vi "OLA.vi"() -> ()   [LabVIEW 2019]
doc: "This is the On-Line Analysis module (OLA).\nThis module receives events from the Target Event Builder (TEB) and processes them. The Q Curve is massaged, gains are divided out, the subtracted and poly subtracted signals are calculated, and an area measurement is made. These results are then sent to the Polarization Display Panel (PDP)."
panel:
  out "data_ready":bool
  out "status":string
  in  "port":u16=10000
  out "Bottom Charge":dbl format="%.6e"
  out "Top Charge":dbl format="%.6e"
  in  "Previous Event":i32
  in  "stop":bool
  out "RF Mod":i32
  out "RF Freq":dbl format="%.3f"
  out "Cal Const":dbl format="%.6f"
  out "Baseline":i32
  out "Raw Signal":dbl[](array[numeric]) format="%.4f"
  out "Event Number":i32
  out "Area":dbl format="%.6f"
  out "Polarization":dbl format="%.2f"
  out "PolySubtracted Signal":dbl[](array[numeric]) format="%.4f"
  out "Polyfit Curve":dbl[](array[numeric]) format="%.4f"
  out "Subtracted Signal":dbl[](array[numeric]) format="%.4f"
  out "Baseline Signal":dbl[](array[numeric]) format="%.6f"
  # "Params over TCP/IP"
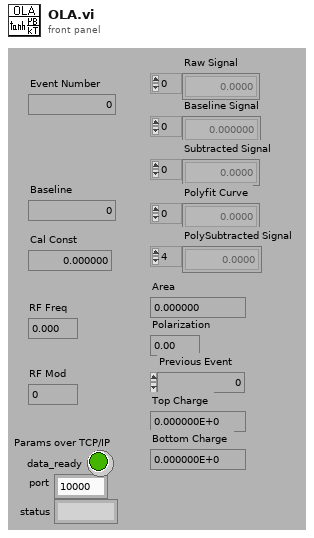
[diagram p1: front panel]
types:
  T1 = enum16{"No Message", "Bad Message", "ClearCharge", "Event=", "Address=", "Ping=", "Stop"}
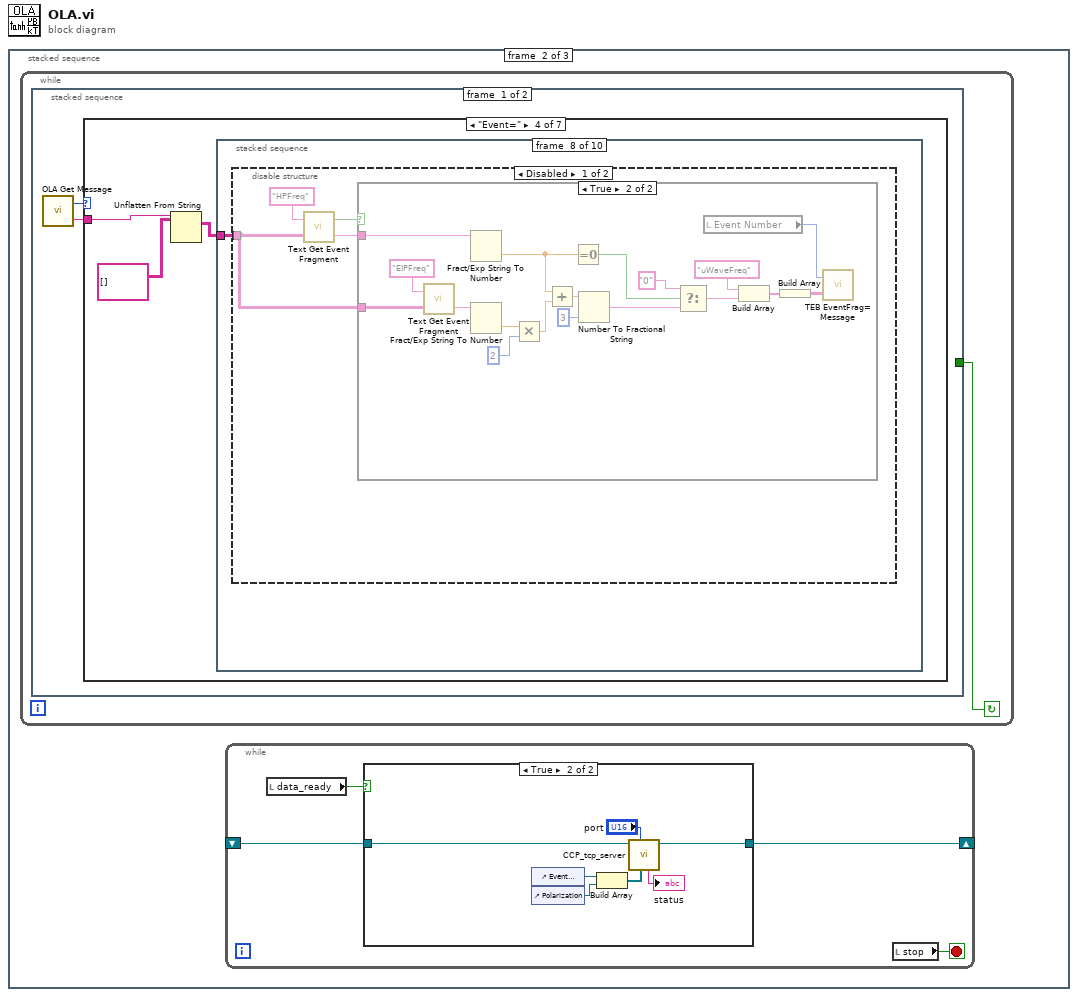
[diagram p0: block diagram]
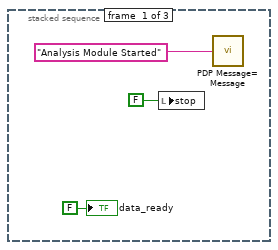
[diagram p2: hidden frame]
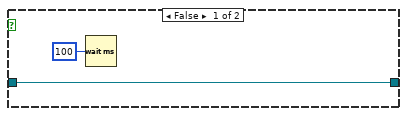
[diagram p3: hidden frame]
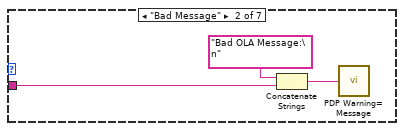
[diagram p5: hidden frame]
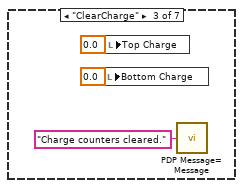
[diagram p6: hidden frame]
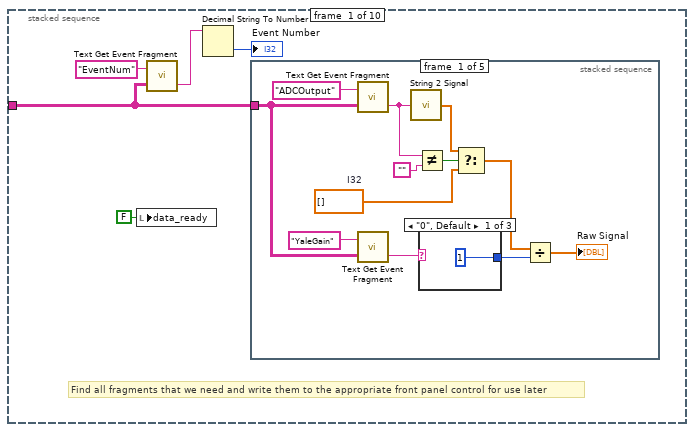
[diagram p7: hidden frame]
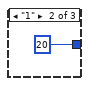
[diagram p8: hidden frame]
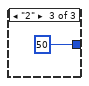
[diagram p9: hidden frame]
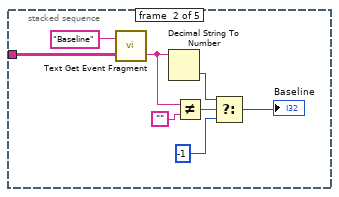
[diagram p10: hidden frame]
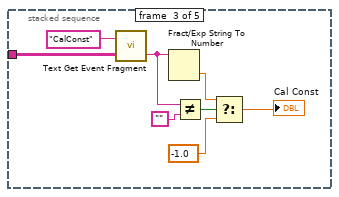
[diagram p11: hidden frame]
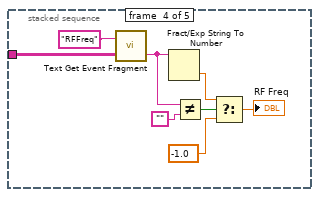
[diagram p12: hidden frame]
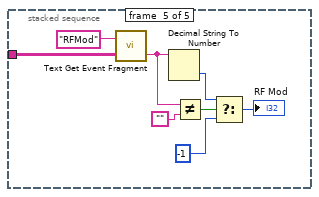
[diagram p13: hidden frame]
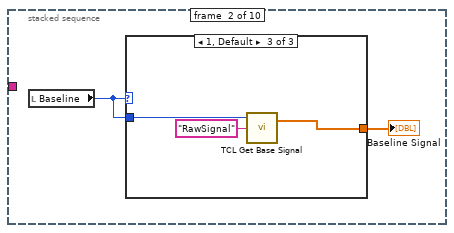
[diagram p14: hidden frame]
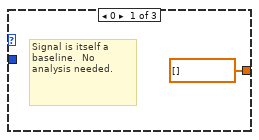
[diagram p15: hidden frame]
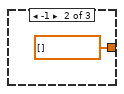
[diagram p16: hidden frame]
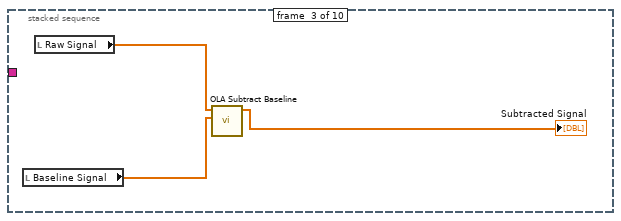
[diagram p17: hidden frame]
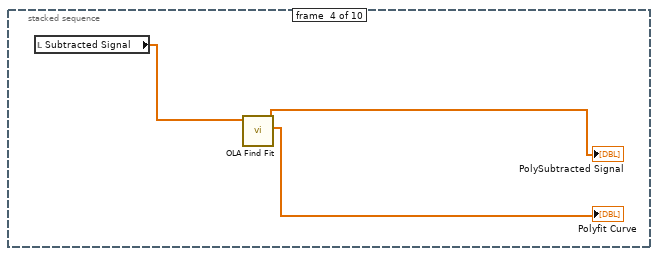
[diagram p18: hidden frame]
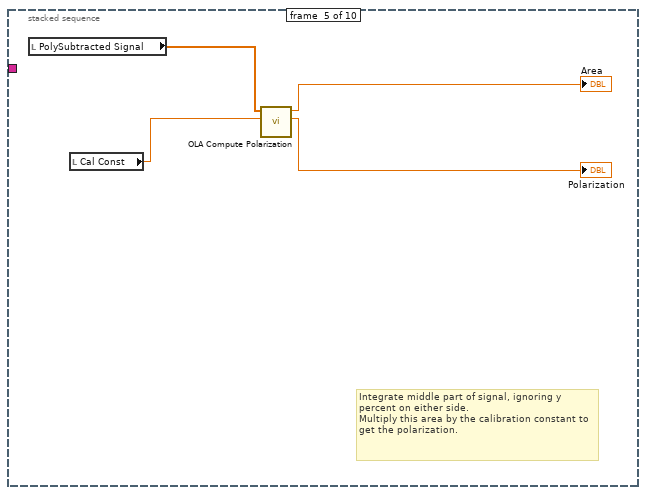
[diagram p19: hidden frame]
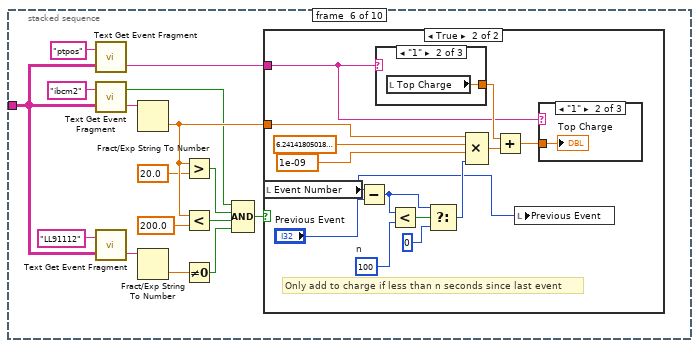
[diagram p20: hidden frame]
diagram:
  n1 = stacked-sequence {
    frame #0 {
      n2 = local write "stop"(FALSE ("stop")) -> ()
      n3 = call "PDP Message= Message.vi"("Message"="Analysis Module Started") -> ()
      "data_ready" <- FALSE ("data_ready")
    }
    frame #1 {
      n4 = while {
        stop <- w17 continue-if-true
        n5 = stacked-sequence {
          tunnel: [_ w238] -> w17
          frame #0 {
            n6 = call "OLA Get Message.vi"() -> ("Text"=w19:string, "OLA Message Type"=w18:T1)
            n7 = case shown="\"Event=\"" w18 {
              tunnel: w19 -> [_ w22 _ w27 w230 w233 _]
              frame "No Message" {
              }
              frame "Bad Message" {
                n8 = Concatenate Strings("Bad OLA Message:\n", w22) -> (w20:string)
                n9 = call "PDP Warning= Message.vi"("Message"=w20) -> ()
              }
              frame "ClearCharge" {
                n10 = local write "Bottom Charge"(0.0 ("Bottom Charge")) -> ()
                n11 = local write "Top Charge"(0.0 ("Top Charge")) -> ()
                n12 = call "PDP Message= Message.vi"("Message"="Charge counters cleared.") -> ()
              }
              frame "Event=" {
                (unwired) FALSE
                n13 = Unflatten From String(type=string[][] [], binary string=w27) -> (value=w26:string[][])  [unwired: 3 in, 2 out]
                n14 = stacked-sequence {
                  tunnel: w26 -> [w30 _ _ _ _ w101 w134 w151 _ _]
                  frame #0 {
                    # "Find all fragments that we need and write them to the appropriate front panel control for use later"
                    n15 = local write "data_ready"(FALSE ("data_ready")) -> ()
                    n16 = call "Text Get Event Fragment.vi"("Event"=w30, "Fragment Type"="EventNum") -> ("Fragment"=w32:string)  [unwired: 1 out]
                    n17 = Decimal String To Number(string=w32) -> (number=→"Event Number":i32)  [unwired: 2 in, 1 out]
                    n18 = stacked-sequence {
                      tunnel: w30 -> [w39 w55 w63 w71 w79]
                      frame #0 {
                        w34 = dbl[] []  # I32
                        n19 = call "Text Get Event Fragment.vi"("Event"=w39, "Fragment Type"="ADCOutput") -> ("Fragment"=w44:string)  [unwired: 1 out]
                        n20 = call "Text Get Event Fragment.vi"("Event"=w39, "Fragment Type"="YaleGain") -> ("Fragment"=w38:string)  [unwired: 1 out]
                        n21 = call "String 2 Signal.vi"("String"=w44) -> ("Signal"=w41:dbl[])
                        n22 = Not Equal?(x=w44, y="") -> (x != y?=w43:bool)
                        n23 = case shown="\"0\", Default" w38 {
                          tunnel: [1 20 50] -> w37
                          frame "0", Default {
                          }
                          frame "1" {
                          }
                          frame "2" {
                          }
                        }
                        n24 = Select(t=w41, s=w43, f=w34) -> (s? t:f=w36:dbl[])
                        n25 = Divide(x=w36, y=w37) -> (x/y=→"Raw Signal":dbl[])
                      }
                      frame #1 {
                        n26 = call "Text Get Event Fragment.vi"("Event"=w55, "Fragment Type"="Baseline") -> ("Fragment"=w50:string)  [unwired: 1 out]
                        n27 = Decimal String To Number(string=w50) -> (number=w53:i32)  [unwired: 2 in, 1 out]
                        n28 = Not Equal?(x=w50, y="") -> (x != y?=w52:bool)
                        n29 = Select(t=w53, s=w52, f=-1) -> (s? t:f=→"Baseline":i32)
                      }
                      frame #2 {
                        n30 = call "Text Get Event Fragment.vi"("Event"=w63, "Fragment Type"="CalConst") -> ("Fragment"=w58:string)  [unwired: 1 out]
                        n31 = Fract/Exp String To Number(string=w58) -> (number=w61:dbl)  [unwired: 3 in, 1 out]
                        n32 = Not Equal?(x=w58, y="") -> (x != y?=w60:bool)
                        n33 = Select(t=w61, s=w60, f=-1.0) -> (s? t:f=→"Cal Const":dbl)
                      }
                      frame #3 {
                        n34 = call "Text Get Event Fragment.vi"("Event"=w71, "Fragment Type"="RFFreq") -> ("Fragment"=w66:string)  [unwired: 1 out]
                        n35 = Fract/Exp String To Number(string=w66) -> (number=w69:dbl)  [unwired: 3 in, 1 out]
                        n36 = Not Equal?(x=w66, y="") -> (x != y?=w68:bool)
                        n37 = Select(t=w69, s=w68, f=-1.0) -> (s? t:f=→"RF Freq":dbl)
                      }
                      frame #4 {
                        n38 = call "Text Get Event Fragment.vi"("Event"=w79, "Fragment Type"="RFMod") -> ("Fragment"=w74:string)  [unwired: 1 out]
                        n39 = Decimal String To Number(string=w74) -> (number=w77:i32)  [unwired: 2 in, 1 out]
                        n40 = Not Equal?(x=w74, y="") -> (x != y?=w76:bool)
                        n41 = Select(t=w77, s=w76, f=-1) -> (s? t:f=→"RF Mod":i32)
                      }
                    }
                  }
                  frame #1 {
                    n42 = local read "Baseline"() -> (w82:i32)
                    n43 = case shown="1, Default" w82 {
                      tunnel: w82 -> [_ _ w87]
                      tunnel: [dbl[] [] ("Baseline") dbl[] [] ("Baseline") w86] -> w81
                      frame 0 {
                        # "Signal is itself a baseline.  No analysis needed."
                      }
                      frame -1 {
                      }
                      frame 1, Default {
                        n44 = call "TCL Get Base Signal.vi"("signal name"="RawSignal", "event number"=w87) -> ("signal"=w86:dbl[])  [unwired: 1 in, 1 out]
                      }
                    }
                    "Baseline Signal" <- w81
                  }
                  frame #2 {
                    n45 = local read "Baseline Signal"() -> (w89:dbl[])
                    n46 = local read "Raw Signal"() -> (w90:dbl[])
                    n47 = call "OLA Subtract Baseline.vi"("baseline"=w89, "raw"=w90) -> ("subtracted"=→"Subtracted Signal":dbl[])  [unwired: 9 in]
                  }
                  frame #3 {
                    n48 = local read "Subtracted Signal"() -> (w93:dbl[])
                    n49 = call "OLA Find Fit.vi"("signal"=w93) -> ("fit"=→"Polyfit Curve":dbl[], "subtracted"=→"PolySubtracted Signal":dbl[])  [unwired: 8 in, 1 out]
                  }
                  frame #4 {
                    # "Integrate middle part of signal, ignoring y percent on either side.\nMultiply this area by the calibration constant to get the polarization."
                    n50 = local read "PolySubtracted Signal"() -> (w97:dbl[])
                    n51 = local read "Cal Const"() -> (w96:dbl)
                    n52 = call "OLA Compute Polarization.vi"("cal"=w96, "signal"=w97) -> ("polarization"=→"Polarization":dbl, "area"=→"Area":dbl)  [unwired: 8 in]
                  }
                  frame #5 {
                    n53 = call "Text Get Event Fragment.vi"("Event"=w101, "Fragment Type"="ptpos") -> ("Fragment"=w99:string)  [unwired: 1 out]
                    n54 = call "Text Get Event Fragment.vi"("Event"=w101, "Fragment Type"="ibcm2") -> ("Fragment"=w110:string, "Found"=w98:bool)
                    n55 = call "Text Get Event Fragment.vi"("Event"=w101, "Fragment Type"="LL91112") -> ("Fragment"=w112:string)  [unwired: 1 out]
                    n56 = Fract/Exp String To Number(string=w110) -> (number=w109:dbl)  [unwired: 3 in, 1 out]
                    n57 = Fract/Exp String To Number(string=w112) -> (number=w111:dbl)  [unwired: 3 in, 1 out]
                    n58 = Greater?(x=w109, y=20.0) -> (0:w104:bool)
                    n59 = Less?(x=w109, y=200.0) -> (x < y?=w106:bool)
                    n60 = Not Equal To 0?(x=w111) -> (x != 0?=w105:bool)
                    n61 = Compound Arithmetic op=AND(w98, w104, w106, w105) -> (w103:bool)
                    n62 = case shown="True" w103 {
                      tunnel: w109 -> [_ w124]
                      tunnel: w99 -> [_ w115]
                      frame False {
                      }
                      frame True {
                        w123 = 100  # n
                        # "Only add to charge if less than n seconds since last event"
                        n63 = local read "Event Number"() -> (w114:i32)
                        n64 = Subtract(x=w114, y="Previous Event") -> (x-y=w120:i32)
                        n65 = case shown="\"1\"" w115 {
                          tunnel: [0.0 w131 w132] -> w117
                          frame "0", Default {
                          }
                          frame "1" {
                            n66 = local read "Top Charge"() -> (w131:dbl)
                          }
                          frame "2" {
                            n67 = local read "Bottom Charge"() -> (w132:dbl)
                          }
                        }
                        n68 = Less?(x=w120, y=w123) -> (x < y?=w121:bool)
                        n69 = Select(t=w120, s=w121, f=0) -> (s? t:f=w118:i32)
                        n70 = Compound Arithmetic op=MULTIPLY(w124, 6.241418050181001e+18, 1e-09 ("Input"), w118) -> (w122:dbl)
                        n71 = Add(x=w117, y=w122) -> (x+y=w116:dbl)
                        n72 = local write "Previous Event"(w114) -> ()
                        n73 = case shown="\"1\"" w115 {
                          tunnel: w116 -> [_ w128 w129]
                          frame "0", Default {
                          }
                          frame "1" {
                            "Top Charge" <- w128
                          }
                          frame "2" {
                            "Bottom Charge" <- w129
                          }
                        }
                      }
                    }
                  }
                  frame #6 {
                    n74 = call "Text Get Event Fragment.vi"("Event"=w134, "Fragment Type"="He4Temp") -> ("Found"=w133:bool)  [unwired: 1 out]
                    n75 = case shown="False" w133 {
                      tunnel: w134 -> [w142 _]
                      frame False {
                        n76 = call "Text Get Event Fragment.vi"("Event"=w142, "Fragment Type"="He4Press") -> ("Fragment"=w150:string)  [unwired: 1 out]
                        n77 = call "Text Get Event Fragment.vi"("Event"=w142, "Fragment Type"="He4Range") -> ("Fragment"=w141:string)  [unwired: 1 out]
                        n78 = Fract/Exp String To Number(string=w150) -> (number=w136:dbl)  [unwired: 3 in, 1 out]
                        n79 = Fract/Exp String To Number(string=w141) -> (number=w140:dbl)  [unwired: 3 in, 1 out]
                        n80 = expression code="10**(-x+2)"(w140) -> (w139:dbl)
                        n81 = Multiply(x=w136, y=w139) -> (x*y=w137:dbl)
                        n82 = call "TTM 4He Press to Temp.vi"("4He Vapor Pressure (torr)"=w137) -> ("4He Temp (K)"=w138:dbl)
                        n83 = Number To Exponential String(number=w138) -> (E-format string=w148:string)  [unwired: 3 in]
                        n84 = local read "Event Number"() -> (w145:i32)
                        n85 = Build Array("He4Temp", w148) -> (w144:string[])
                        n86 = Build Array(w144) -> (w146:string[][])
                        n87 = call "TEB EventFrag= Message.vi"("Event Fragment(s)"=w146, "Event Number"=w145) -> ()
                      }
                      frame True {
                      }
                    }
                  }
                  frame #7 {
                    n88 = disable-structure shown="Disabled" {
                      disable-tunnel: w151 -> [w154 _]
                      frame Disabled {
                        n89 = call "Text Get Event Fragment.vi"("Event"=w154, "Fragment Type"="HPFreq") -> ("Fragment"=w152:string, "Found"=w153:bool)
                        n90 = case shown="True" w153 {
                          tunnel: w154 -> [w157 w175]
                          tunnel: w152 -> [_ w172]
                          frame False {
                            n91 = call "Text Get Event Fragment.vi"("Event"=w157, "Fragment Type"="EIPFreq") -> ("Fragment"=w156:string)  [unwired: 1 out]
                            n92 = local read "Event Number"() -> (w159:i32)
                            n93 = Build Array("uWaveFreq", w156) -> (w158:string[])
                            n94 = Build Array(w158) -> (w160:string[][])
                            n95 = call "TEB EventFrag= Message.vi"("Event Fragment(s)"=w160, "Event Number"=w159) -> ()
                          }
                          frame True {
                            n96 = call "Text Get Event Fragment.vi"("Event"=w175, "Fragment Type"="EIPFreq") -> ("Fragment"=w174:string)  [unwired: 1 out]
                            n97 = Fract/Exp String To Number(string=w172) -> (number=w165:dbl)  [unwired: 3 in, 1 out]
                            n98 = Fract/Exp String To Number(string=w174) -> (number=w173:dbl)  [unwired: 3 in, 1 out]
                            n99 = Multiply(x=w173, y=2) -> (x*y=w171:dbl)
                            n100 = Add(x=w165, y=w171) -> (x+y=w170:dbl)
                            n101 = Equal To 0?(x=w165) -> (x = 0?=w164:bool)
                            n102 = Number To Fractional String(number=w170, precision (6)=i16 3) -> (F-format string=w166:string)  [unwired: 2 in]
                            n103 = Select(t="0", s=w164, f=w166) -> (s? t:f=w167:string)
                            n104 = local read "Event Number"() -> (w177:i32)
                            n105 = Build Array("uWaveFreq", w167) -> (w176:string[])
                            n106 = Build Array(w176) -> (w178:string[][])
                            n107 = call "TEB EventFrag= Message.vi"("Event Fragment(s)"=w178, "Event Number"=w177) -> ()
                          }
                        }
                      }
                      frame Enabled {
                      }
                    }
                  }
                  frame #8 {
                    w183 = string[] [] ("Array Constant")
                    # "Ship all results off to the event builder."
                    n108 = local read "PolySubtracted Signal"() -> (w181:dbl[])
                    n109 = local read "Bottom Charge"() -> (w193:dbl)
                    n110 = local read "Subtracted Signal"() -> (w218:dbl[])
                    n111 = local read "Polyfit Curve"() -> (w217:dbl[])
                    n112 = local read "Polarization"() -> (w204:dbl)
                    n113 = local read "Baseline Signal"() -> (w223:dbl[])
                    n114 = local read "Top Charge"() -> (w194:dbl)
                    n115 = local read "Raw Signal"() -> (w201:dbl[])
                    n116 = local read "Area"() -> (w212:dbl)
                    n117 = Array Size(array=w181) -> (size(s)=w182:i32)
                    n118 = Equal To 0?(x=w182) -> (x = 0?=w184:bool)
                    n119 = call "Signal 2 String.vi"("Signal"=w201) -> ("String"=w202:string)
                    n120 = call "Signal 2 String.vi"("Signal"=w223) -> ("String"=w222:string)
                    n121 = call "Signal 2 String.vi"("Signal"=w218) -> ("String"=w219:string)
                    n122 = call "Signal 2 String.vi"("Signal"=w217) -> ("String"=w216:string)
                    n123 = call "Signal 2 String.vi"("Signal"=w181) -> ("String"=w213:string)
                    n124 = Number To Exponential String(number=w194) -> (E-format string=w196:string)  [unwired: 3 in]
                    n125 = Number To Exponential String(number=w193) -> (E-format string=w191:string)  [unwired: 3 in]
                    n126 = Number To Exponential String(number=w204) -> (E-format string=w205:string)  [unwired: 3 in]
                    n127 = Number To Exponential String(number=w212) -> (E-format string=w211:string)  [unwired: 3 in]
                    n128 = Build Array("RawSignal", w202) -> (w200:string[])
                    n129 = Build Array("BaseSignal", w222) -> (w199:string[])
                    n130 = Build Array("SubSignal", w219) -> (w198:string[])
                    n131 = Build Array("PolyCurve", w216) -> (w197:string[])
                    n132 = Build Array("PolySignal", w213) -> (w209:string[])
                    n133 = Build Array("TopCharge", w196) -> (w190:string[])
                    n134 = Build Array("BottomCharge", w191) -> (w189:string[])
                    n135 = Build Array("Polarization", w205) -> (w188:string[])
                    n136 = Build Array("Area", w211) -> (w187:string[])
                    n137 = Select(t=w183, s=w184, f=w188) -> (s? t:f=w185:string[])
                    n138 = Select(t=w183, s=w184, f=w187) -> (s? t:f=w186:string[])
                    n139 = local read "Event Number"() -> (w207:i32)
                    n140 = Build Array(w200, w199, w198, w197, w209, w190, w189, w185, w186) -> (w208:string[][])
                    n141 = call "TEB EventFrag= Message.vi"("Event Fragment(s)"=w208, "Event Number"=w207) -> ()
                  }
                  frame #9 {
                    # "Tell event builder we're done processing this event."
                    n142 = local read "Event Number"() -> (w226:i32)
                    n143 = local write "data_ready"(TRUE ("data_ready")) -> ()
                    n144 = call "TEB Processed= Message.vi"("Module Name"="OLA", "Event Number"=w226) -> ()
                  }
                }
              }
              frame "Address=" {
                n145 = Scan From String(format string="%s,%[.0-9]:%d" ("Format String"), input string=w230) -> (output 1=w228:string, output 2=w229:string, output 3=w227:i32)  [unwired: 5 in, 3 out]
                n146 = call "Message Set Module Address.vi"("Port"=w227, "Address"=w229, "Module"=w228) -> ()
              }
              frame "Ping=" {
                n147 = Get Date/Time In Seconds() -> (seconds since 1Jan1904=w232:timestamp)
                n148 = To Double Precision Float(number=w232) -> (double precision float=w235:dbl)
                n149 = Format Into String(format string="PingResponse=OLA,%.0f", w235) -> (resulting string=w234:string)  [unwired: 2 in, 1 out]
                n150 = call "Message Send.vi"("Message"=w234, "Destination"=w233) -> ()
              }
              frame "Stop" {
                n151 = local write "stop"(TRUE ("stop")) -> ()
              }
            }
          }
          frame #1 {
            n152 = Not(x="stop") -> (.not. x?=w238:bool)
          }
        }
      }
      n153 = while {
        shift-right: [w5] -> _
        shift-left: _ -> [w6]
        stop <- w7 stop-if-true
        n154 = local read "data_ready"() -> (w4:bool)
        n155 = case shown="True" w4 {
          tunnel: w6 -> [w9 w16]
          tunnel: [w9 w15] -> w5
          frame False {
            n156 = Wait (ms)(milliseconds to wait=u32 100) -> ()  [unwired: 1 out]
          }
          frame True {
            n157 = control-ref of="Event Number"() -> (w11:refnum<vi>)
            n158 = control-ref of="Polarization"() -> (w14:refnum<vi>)
            n159 = Build Array(w11, w14) -> (w10:refnum<vi>[])
            n160 = call "CCP_tcp_server.vi"("value"=w10, "port"="port", "conn_id_in"=w16) -> ("conn_id_out"=w15:refnum<k5>, "status"=→"status":string)  [unwired: 6 in, 1 out]
          }
        }
        n161 = local read "stop"() -> (w7:bool)
      }
    }
    frame #2 {
      n162 = local write "stop"(FALSE ("stop")) -> ()
      n163 = call "PDP Message= Message.vi"("Message"="OLA Module Stopped") -> ()
    }
  }
